vi "Setting2.vi"() -> ()   [LabVIEW 2015]
uses:
  0.Control/Setting_Control_Main Action.ctl
  0.Control/Setting_Control_Pattern Paremeter.ctl
  <vilib>/vision/Measure.llb/Edge Options.ctl
  <vilib>/vision/Measure.llb/Edge Polarity.ctl
  <vilib>/Utility/miscctls.llb/LVPointTypeDef.ctl
  <vilib>/Utility/miscctls.llb/LVBoundsTypeDef.ctl
  <vilib>/userdefined/High Color/IMAQdx.ctl
  <vilib>/vision/NI_Vision_Development_Module.lvlib
panel:
  out "距離(中心到邊)":dbl
  out "間距":sgl
  out "String":string
  out "彈簧距離":sgl
  out "彈簧角度":sgl
  out "塑膠蓋角度":sgl
  out "Pattern":T1(plugin-control)
  in  "相機、光源":T2 {"光源亮度" step=1 scale=0.0..255.0; "相機選擇" items=["相機 1", "相機 2"]; "光源選擇" items=["光源 1", "光源 2"]}
  out "Image":T1(plugin-control)
  in  "Tab Control":enum32{"設定", "Match參數", "找邊參數", "間距參數"}(tab)
  in  "單步測試":bool
  in  "連續測試":bool
  in  "檢測項目塑膠蓋":enum16{"Pattern", "Match", "找邊", "間距"}(ring)
  in  "取像":bool
  in  "連續取像":bool
  in  "離開":bool
  in  "匯入圖片":bool
  in  "確認檢測項目":bool
  in  "樣本比對參數L":T3={"方法"=1, "分數"=800.0, "起始角度"=-5.0, "結束角度"=5.0} {"結束角度" min=-180 max=180 step=5; "方法" items=["快速比對"=1, "精準比對"=2]; "起始角度" min=-180 max=180 step=5}
  in  "pattern_Angle Range":cluster{"Start Angle":sgl, "End Angle":sgl}={"Start Angle"=180.0, "End Angle"=-180.0}
  in  "Scan Direction":u16(ring) items=["Left To Right", "Right To Left", "Top To Bottom", "Bottom To Top"]
  in  "Edge Options":T4={"Edge Polarity"=0, "Kernel Size"=3, "Width"=3, "Minimum Edge Strength"=10.0, "Interpolation Type"=enum."Bilinear Fixed", "Data Processing Method"=enum."Average"} {"Edge Polarity" items=["All Edges", "Rising Edges", "Falling Edges"]; "Minimum Edge Strength" format="%.2f"; "Width" step=2; "Kernel Size" step=2}
  in  "setting":T6={"Contrast"=40, "Filter width"=4, "Steepness"=2, "Subsampling Ratio"=5}
  out "Set action":T7
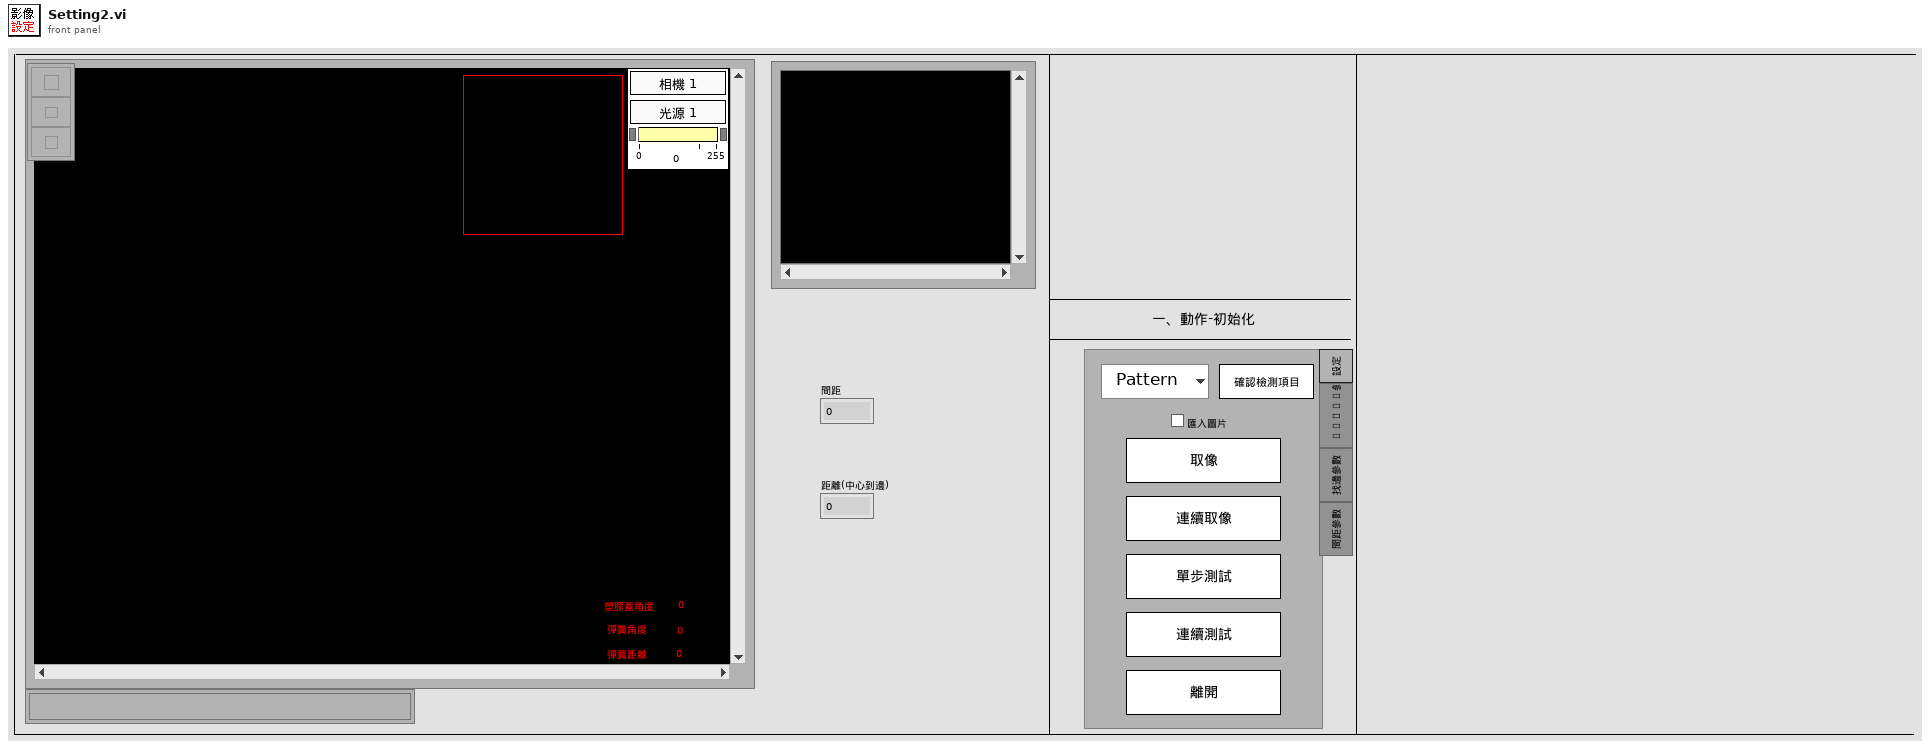
[diagram p1: front panel]
types:
  T1 = typedef "IMAQ Image.ctl" = refnum<image>
  T2 = typedef "Control_Camera&Light.ctl" = cluster{"相機選擇":u8, "光源選擇":u16, "光源亮度":u8}
  T3 = typedef "Setting_Control_Pattern Paremeter.ctl" = cluster{"方法":u16, "分數":sgl, "起始角度":sgl, "結束角度":sgl}
  T4 = typedef "Edge Options.ctl" = cluster{"Edge Polarity":T5, "Kernel Size":u32, "Width":u32, "Minimum Edge Strength":sgl, "Interpolation Type":enum32{"Zero Order", "Bilinear", "Quadratic", "Cubic", "Bilinear Fixed"}, "Data Processing Method":enum32{"Average", "Median"}}
  T5 = typedef "Edge Polarity.ctl" = u32
  T6 = cluster{"Contrast":i32, "Filter width":i32, "Steepness":i32, "Subsampling Ratio":u32}
  T7 = typedef "Setting_Control_Main Action.ctl" = enum16{"一、動作-初始化", "二、動作-單次取像", "三、動作-連續取像", "四、動作-單步測試", "五、動作-連續測試", "六、動作-離開", "1.0 功能-IO控制", "       1.1 IO-初始化", "       1.2 Set Point(EOT On)", "       1.3Set Point(EOT Off)", "       1.4Get Point(SOT)", "2.0功能-相機控制", "       2.1相機-初始化", "       2.2相機-取像", "       2.3相機-關閉", "3.0功能-影像控制", "       3.1影像-初始化", "       3.2影像-更新影像", "       3.3影像-儲存影像", "4.0功能-檢測", "       4.1檢測-初始化", "      4.2浪代-浪代", "             4.2.1浪代-Pattern", "             4.2.2浪代-Match", "             4.2.3檢測-找邊", "             4.2.4檢測-間距", "5.0功能-檔案", "       5.1檔案-初始化", "       5.2檔案-儲存檔案", "       5.3檔案-開啟檔案", "       5.4檔案-匯入檔案", "6.0 錯誤", "7.0等待", "       7.1等待(計算時間)", "8.0離開", "9.0功能-機台驗證", "      9.1機台驗證-初始化", "      9.2機台驗證-檢測", "10.0對話視窗", "11.光源控制", "       11.1光源控制-初始化", "       11.2光源控制-光源開啟", "       11.3光源控制-光源關閉", "       11.4光源控制-通訊關閉"}
  T8 = typedef "LVPointTypeDef.ctl" = cluster{"Horizontal":i16, "Vertical":i16}
  T9 = typedef "IMAQdx.ctl" = refnum<k21>
  T10 = typedef "action_camera.ctl" = enum16{"初始化", "取像", "匯入影像", "結束"}
  T11 = typedef "Control_Indicator Action(FGV).ctl" = enum16{"Set Data", "Get Data", "Idle"}
  T12 = typedef "Image action.ctl" = enum16{"初始化", "創造記憶體", "寫入圖片", "讀取圖片", "刪除圖片", "等待"}
  T13 = typedef "LVBoundsTypeDef.ctl" = cluster{"Width":u32, "Height":u32}
  T14 = typedef "IMAQ Coordinate System" = cluster{"Reference System":cluster{"Origin":cluster{"X":sgl, "Y":sgl}, "Angle (deg)":sgl, "Axis Reference":u32}, "Measurement System":cluster{"Origin":cluster{"X":sgl, "Y":sgl}, "Angle (deg)":sgl, "Axis Reference":u32}}
  T15 = cluster{"樣本比對參數L":T3, "ROI":cluster{"Global Rectangle":i32[], "Contours":cluster{"Contour Type":u32, "ROI Type":u32, "Points":i32[]}[]}, "Coordinate System Out":T14}
  T16 = typedef "Action_Data.ctl" = enum16{"Initialize", "Get Data", "Set Data", "Delete Data", "Idle"}
  T17 = cluster{"setting":cluster{"Contrast":i32, "Filter width":i32, "Steepness":i32, "Subsampling Ratio":u32}, "ROI":cluster{"Global Rectangle":i32[], "Contours":cluster{"Contour Type":u32, "ROI Type":u32, "Points":i32[]}[]}}
  T18 = cluster{"Scan Direction":u16, "ROI":cluster{"Global Rectangle":i32[], "Contours":cluster{"Contour Type":u32, "ROI Type":u32, "Points":i32[]}[]}, "Edge Options":T4}
  T19 = typedef "Control_Indicator(FGV) #.ctl" = cluster{"相機、光源":cluster{"相機選擇":u8, "光源選擇":u16, "光源亮度":u8}, "Session Out":T9, "Cam#Light#Strength":string}
  T20 = typedef "光源通訊_action_control.ctl" = enum16{"initial", "開啟光源", "關閉光源", "close"}
  T21 = typedef "Image Type" = u32
  T22 = cluster{"Global Rectangle":i32[], "Contours":cluster{"Contour Type":u32, "ROI Type":u32, "Points":i32[]}[]}
  T23 = cluster{"Position":cluster{"x":sgl, "y":sgl}, "Angle":sgl, "Scale":sgl, "Score":sgl, "Bounding Box":cluster{"x":sgl, "y":sgl}[]}[]
  T24 = cluster{"Position":cluster{"x":sgl, "y":sgl}, "Angle":sgl, "Scale":sgl, "Score":sgl, "Bounding Box":cluster{"x":sgl, "y":sgl}[]}
  T25 = cluster{"Center (Pixels)":cluster{"X":sgl, "Y":sgl}, "Radius (Pixels)":dbl, "Center (Real-World)":cluster{"X":sgl, "Y":sgl}, "Radius (Real-World)":dbl, "Roundness (Real-World)":dbl, "Average Strength":dbl, "Average SNR (dB)":dbl}
  T26 = cluster{"Search  Direction":u32, "Edge Options":T4, "Show Search Area":bool, "Show Search Lines":bool, "Show Edges Found":bool, "Show Result":bool, "Search Area Color":u32, "Search Lines Color":u32, "Edge Locations Color":u32, "Result Color":u32, "Overlay Group Name":string}
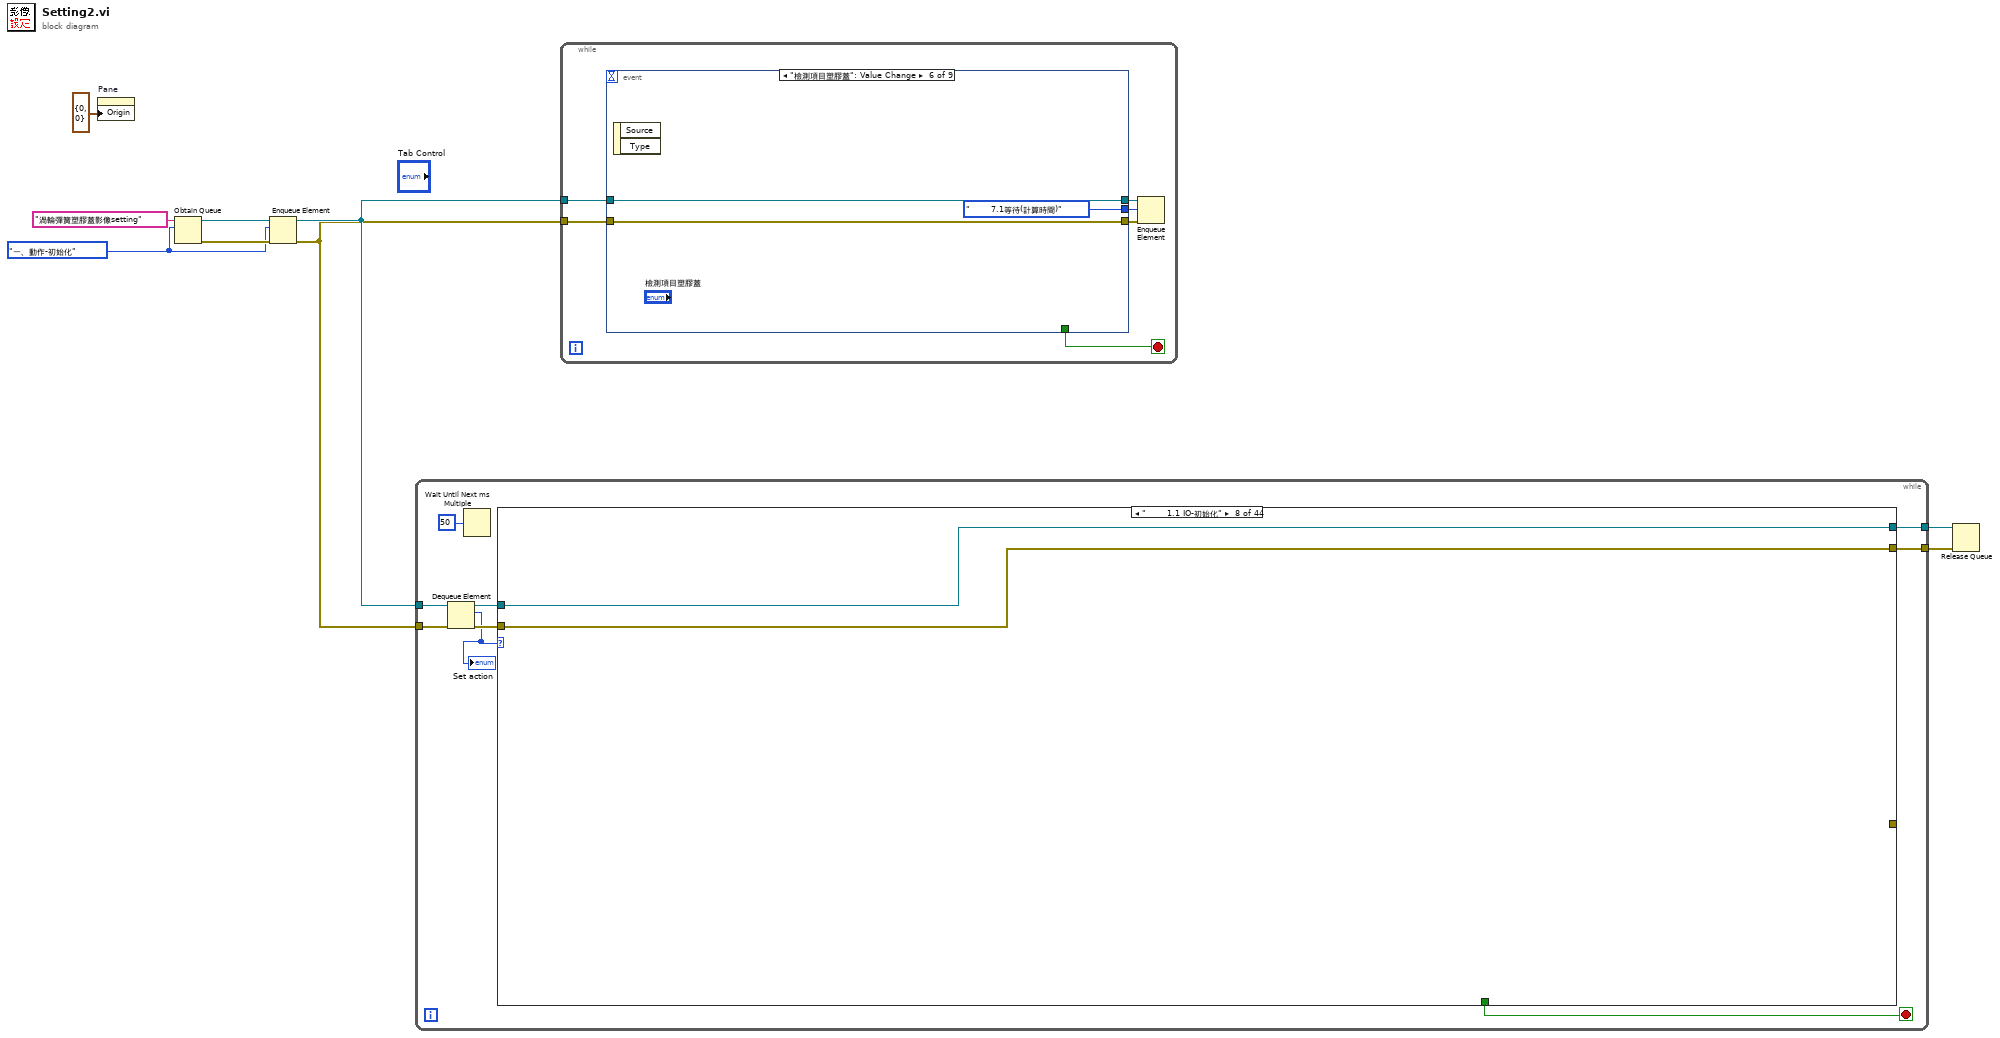
[diagram p0: block diagram]
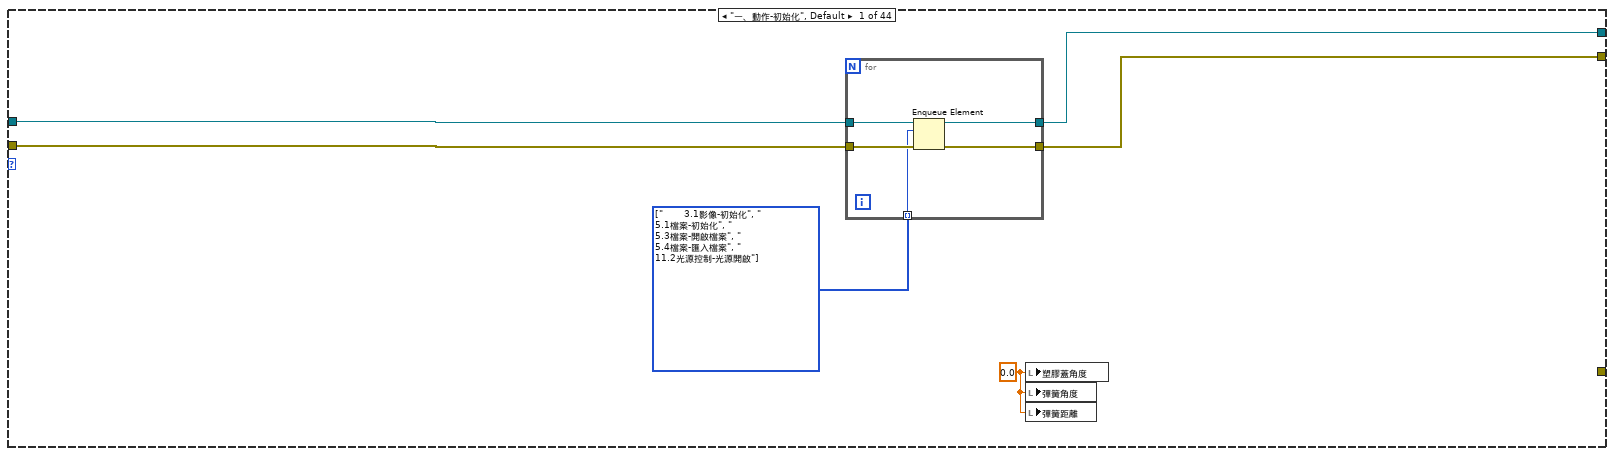
[diagram p2: hidden frame]
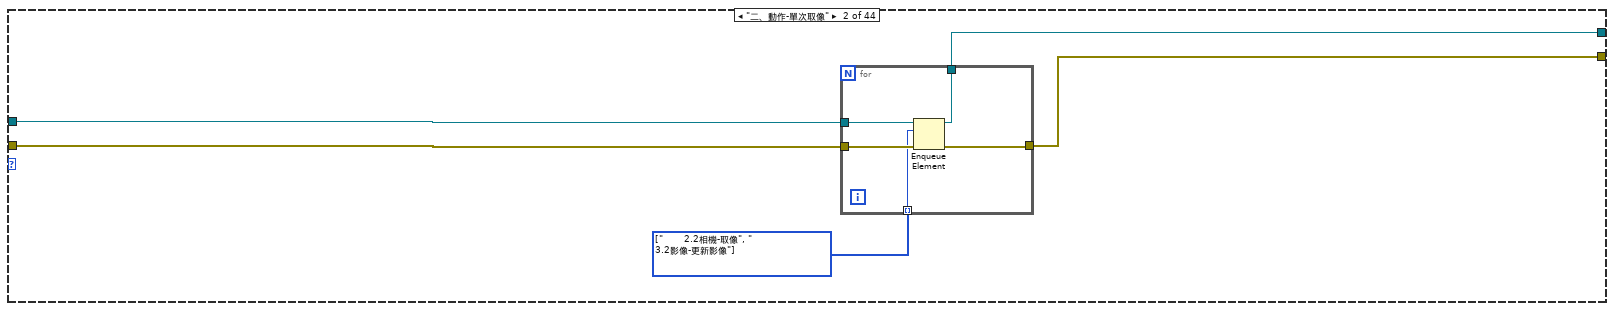
[diagram p3: hidden frame]
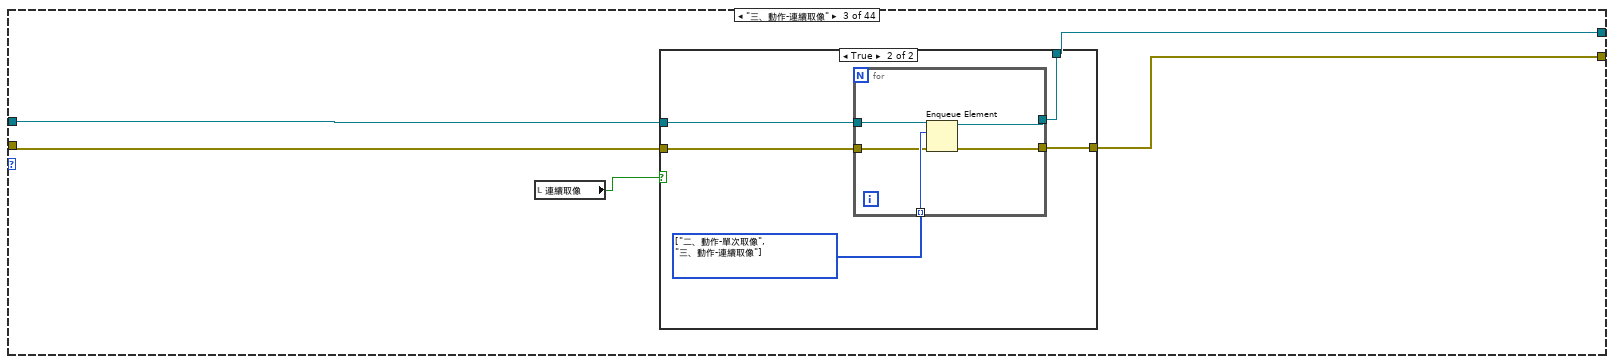
[diagram p4: hidden frame]
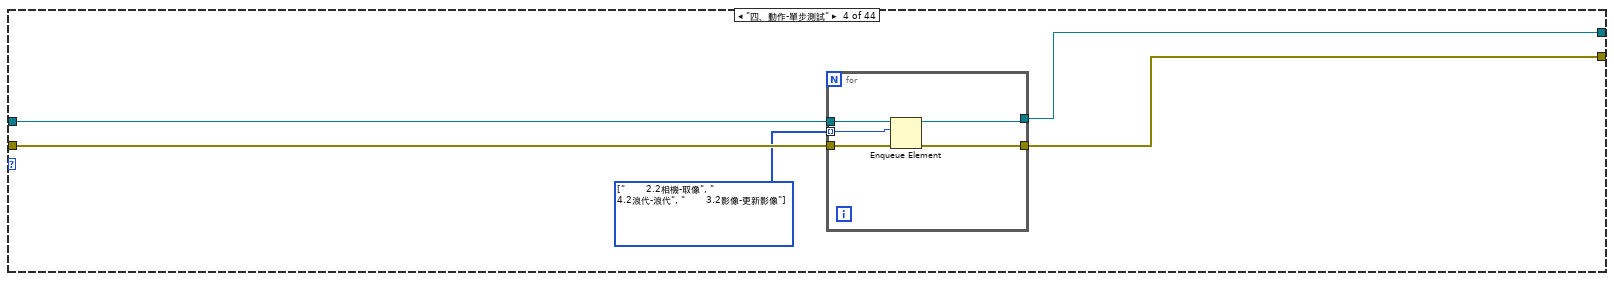
[diagram p6: hidden frame]
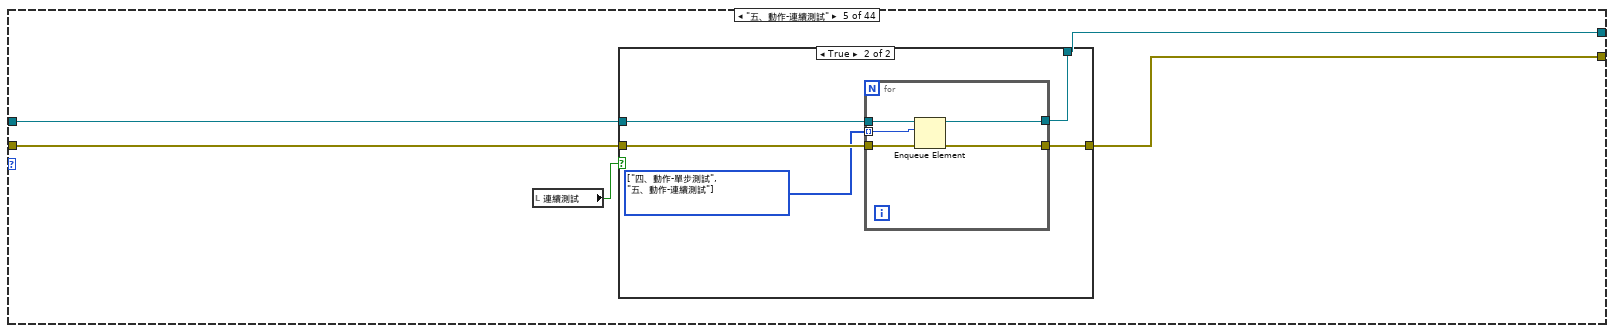
[diagram p7: hidden frame]
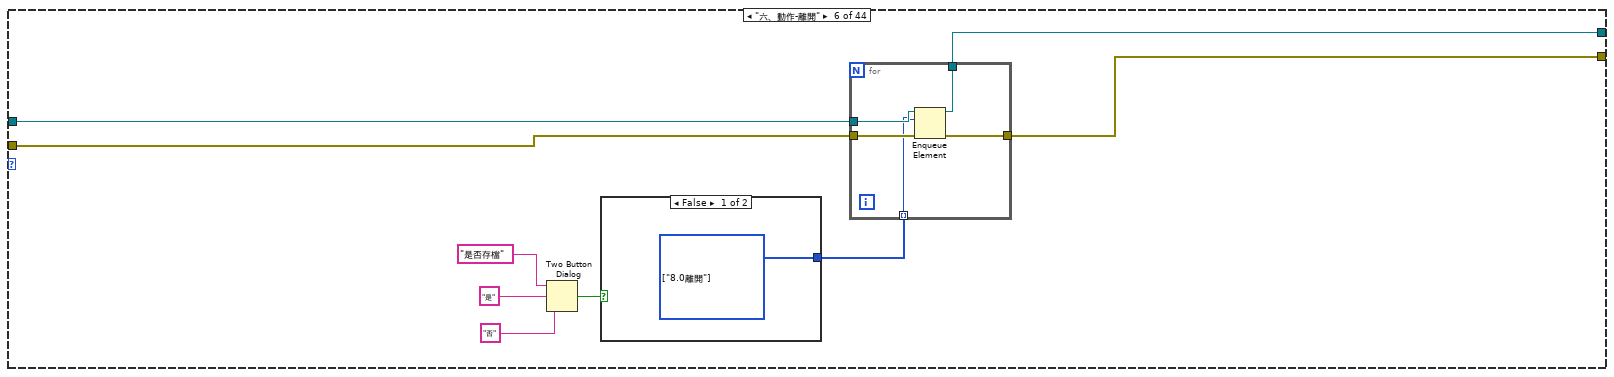
[diagram p9: hidden frame]
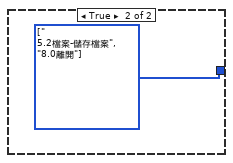
[diagram p10: hidden frame]
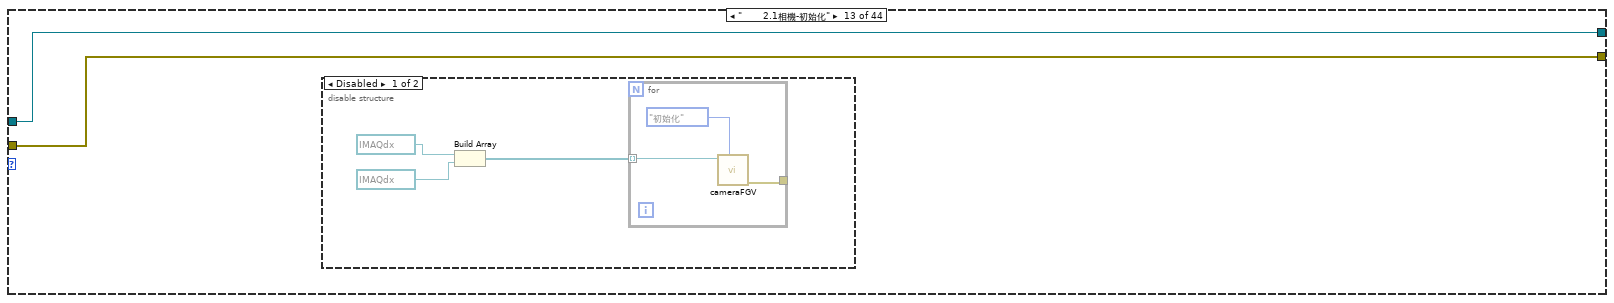
[diagram p16: hidden frame]
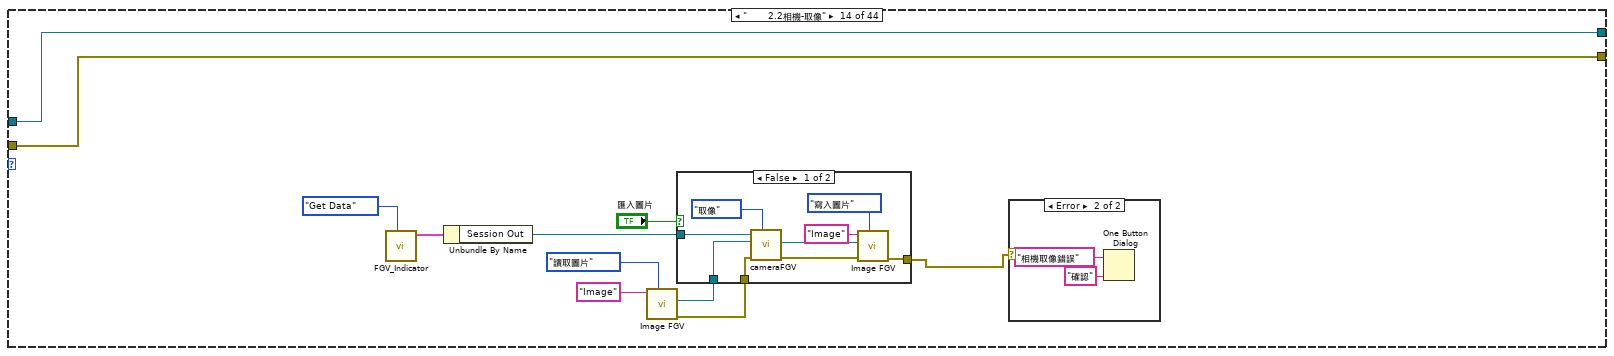
[diagram p18: hidden frame]
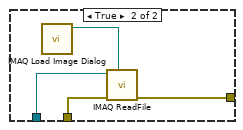
[diagram p20: hidden frame]
diagram:
  w3 = Setting_Control_Main_Action."一、動作-初始化" ("Set action")
  n1 = property on="Pane" class="Pane"("Origin"=T8 {"Horizontal"=0, "Vertical"=0}) -> ()  [unwired: 2 in, 2 out]
  n2 = Obtain Queue(name (unnamed)="渦輪彈簧塑膠蓋影像setting", element data type=w3) -> (queue out=w8:refnum<queue>, error out=w7:errorcluster)  [unwired: 3 in, 1 out]
  n3 = Enqueue Element(queue=w8, element=w3, error in (no error)=w7) -> (queue out=w6:refnum<queue>, error out=w5:errorcluster)  [unwired: 1 in, 1 out]
  n4 = while {
    tunnel: w6 -> [w18]
    tunnel: w5 -> [w17]
    tunnel: [w11] -> w2
    tunnel: [w10] -> w1
    stop <- w16 stop-if-true
    n5 = Dequeue Element(queue=w18, error in (no error)=w17) -> (queue out=w15:refnum<queue>, element=w12:T7, error out=w14:errorcluster)  [unwired: 1 in, 1 out]
    "Set action" <- w12
    n6 = Wait Until Next ms Multiple(millisecond multiple=u32 50) -> ()  [unwired: 1 out]
    n7 = case shown="\"       1.1 IO-初始化\"" w12 {
      tunnel: [_ _ _ _ _ _ _ _ _ _ _ _ _ _ _ _ _ _ _ _ _ _ _ _ _ _ _ _ _ _ _ _ _ _ TRUE _ _ _ _ _ _ _ _ _] -> w16
      tunnel: w15 -> [w21 w34 w44 w61 w71 w92 w101 w103 w105 w107 w109 w111 w113 w126 w147 w155 w160 w183 w188 w190 w192 w195 w357 w381 w409 w435 w448 w451 w474 w493 w564 w579 w581 w583 w586 w588 w590 w592 w594 w596 w598 w612 w624 w628]
      tunnel: w14 -> [w24 w33 w43 w60 w70 w91 w100 w102 w104 w106 w108 w110 w112 w121 w146 w154 w158 w177 w187 w189 w191 w194 w355 w379 w408 w434 w447 w449 w473 w492 w563 w578 w580 w582 w585 w587 w589 w591 w593 w595 w597 w611 w623 w627]
      tunnel: [w22 w31 w42 w59 w69 w90 w101 w103 w105 w107 w109 w111 w113 w126 w147 w155 w160 w183 w188 w190 w192 w195 w356 w380 w407 w433 w448 w451 w474 w494 w564 w579 w581 w583 w586 w588 w590 w592 w594 w596 w598 w612 w624 w628] -> w11
      tunnel: [w23 w32 w41 w58 w68 w89 w100 w102 w104 w106 w108 w110 w112 w121 w146 w154 w157 w175 w187 w189 w191 w194 w354 w378 w406 w432 w447 w449 w473 w491 w563 w578 w580 w582 w585 w587 w589 w591 w593 w595 w597 w611 w623 w627] -> w10
      tunnel: [_ _ _ _ _ _ _ _ _ _ _ _ _ _ _ _ _ _ _ _ _ w193 _ _ _ _ _ _ _ w489 _ _ _ _ _ _ _ _ _ _ _ _ _ _] -> _
      frame "一、動作-初始化", Default {
        w19 = sgl 0.0 ("塑膠蓋角度")
        w20 = T7[] [enum."       3.1影像-初始化", enum."       5.1檔案-初始化", enum."       5.3檔案-開啟檔案", enum."       5.4檔案-匯入檔案", enum."       11.2光源控制-光源開啟"] items=["一、動作-初始化", "二、動作-單次取像", "三、動作-連續取像", "四、動作-單步測試", "五、動作-連續測試", "六、動作-離開", "1.0 功能-IO控制", "       1.1 IO-初始化", "       1.2 Set Point(EOT On)", "       1.3Set Point(EOT Off)", "       1.4Get Point(SOT)", "2.0功能-相機控制", "       2.1相機-初始化", "       2.2相機-取像", "       2.3相機-關閉", "3.0功能-影像控制", "       3.1影像-初始化", "       3.2影像-更新影像", "       3.3影像-儲存影像", "4.0功能-檢測", "       4.1檢測-初始化", "      4.2浪代-浪代", "             4.2.1浪代-Pattern", "             4.2.2浪代-Match", "             4.2.3檢測-找邊", "             4.2.4檢測-間距", "5.0功能-檔案", "       5.1檔案-初始化", "       5.2檔案-儲存檔案", "       5.3檔案-開啟檔案", "       5.4檔案-匯入檔案", "6.0 錯誤", "7.0等待", "       7.1等待(計算時間)", "8.0離開", "9.0功能-機台驗證", "      9.1機台驗證-初始化", "      9.2機台驗證-檢測", "10.0對話視窗", "11.光源控制", "       11.1光源控制-初始化", "       11.2光源控制-光源開啟", "       11.3光源控制-光源關閉", "       11.4光源控制-通訊關閉"]
        n8 = for {
          tunnel: w21 -> [w29]
          tunnel: w24 -> [w28]
          tunnel: [w27] -> w23
          tunnel: [w26] -> w22
          tunnel: w20 -> [w25] mode=indexing
          n9 = Enqueue Element(queue=w29, element=w25, error in (no error)=w28) -> (queue out=w26:refnum<queue>, error out=w27:errorcluster)  [unwired: 1 in, 1 out]
        }
        n10 = local write "塑膠蓋角度"(w19) -> ()
        n11 = local write "彈簧角度"(w19) -> ()
        n12 = local write "彈簧距離"(w19) -> ()
      }
      frame "二、動作-單次取像" {
        w30 = T7[] [enum."       2.2相機-取像", enum."       3.2影像-更新影像"] items=["一、動作-初始化", "二、動作-單次取像", "三、動作-連續取像", "四、動作-單步測試", "五、動作-連續測試", "六、動作-離開", "1.0 功能-IO控制", "       1.1 IO-初始化", "       1.2 Set Point(EOT On)", "       1.3Set Point(EOT Off)", "       1.4Get Point(SOT)", "2.0功能-相機控制", "       2.1相機-初始化", "       2.2相機-取像", "       2.3相機-關閉", "3.0功能-影像控制", "       3.1影像-初始化", "       3.2影像-更新影像", "       3.3影像-儲存影像", "4.0功能-檢測", "       4.1檢測-初始化", "      4.2浪代-浪代", "             4.2.1浪代-Pattern", "             4.2.2浪代-Match", "             4.2.3檢測-找邊", "             4.2.4檢測-間距", "5.0功能-檔案", "       5.1檔案-初始化", "       5.2檔案-儲存檔案", "       5.3檔案-開啟檔案", "       5.4檔案-匯入檔案", "6.0 錯誤", "7.0等待", "       7.1等待(計算時間)", "8.0離開", "9.0功能-機台驗證", "      9.1機台驗證-初始化", "      9.2機台驗證-檢測", "10.0對話視窗", "11.光源控制", "       11.1光源控制-初始化", "       11.2光源控制-光源開啟", "       11.3光源控制-光源關閉", "       11.4光源控制-通訊關閉"]
        n13 = for {
          tunnel: w34 -> [w39]
          tunnel: w33 -> [w38]
          tunnel: [w37] -> w32
          tunnel: [w36] -> w31
          tunnel: w30 -> [w35] mode=indexing
          n14 = Enqueue Element(queue=w39, element=w35, error in (no error)=w38) -> (queue out=w36:refnum<queue>, error out=w37:errorcluster)  [unwired: 1 in, 1 out]
        }
      }
      frame "三、動作-連續取像" {
        n15 = local read "連續取像"() -> (w40:bool)
        n16 = case shown="True" w40 {
          tunnel: w44 -> [w46 w50]
          tunnel: w43 -> [w45 w49]
          tunnel: [w46 w48] -> w42
          tunnel: [w45 w47] -> w41
          frame False {
          }
          frame True {
            w51 = T7[] [enum."二、動作-單次取像", enum."三、動作-連續取像"] items=["一、動作-初始化", "二、動作-單次取像", "三、動作-連續取像", "四、動作-單步測試", "五、動作-連續測試", "六、動作-離開", "1.0 功能-IO控制", "       1.1 IO-初始化", "       1.2 Set Point(EOT On)", "       1.3Set Point(EOT Off)", "       1.4Get Point(SOT)", "2.0功能-相機控制", "       2.1相機-初始化", "       2.2相機-取像", "       2.3相機-關閉", "3.0功能-影像控制", "       3.1影像-初始化", "       3.2影像-更新影像", "       3.3影像-儲存影像", "4.0功能-檢測", "       4.1檢測-初始化", "      4.2浪代-浪代", "             4.2.1浪代-Pattern", "             4.2.2浪代-Match", "             4.2.3檢測-找邊", "             4.2.4檢測-間距", "5.0功能-檔案", "       5.1檔案-初始化", "       5.2檔案-儲存檔案", "       5.3檔案-開啟檔案", "       5.4檔案-匯入檔案", "6.0 錯誤", "7.0等待", "       7.1等待(計算時間)", "8.0離開", "9.0功能-機台驗證", "      9.1機台驗證-初始化", "      9.2機台驗證-檢測", "10.0對話視窗", "11.光源控制", "       11.1光源控制-初始化", "       11.2光源控制-光源開啟", "       11.3光源控制-光源關閉", "       11.4光源控制-通訊關閉"]
            n17 = for {
              tunnel: [w56] -> w47
              tunnel: [w55] -> w48
              tunnel: w51 -> [w54] mode=indexing
              tunnel: w50 -> [w53]
              tunnel: w49 -> [w52]
              n18 = Enqueue Element(queue=w53, element=w54, error in (no error)=w52) -> (queue out=w55:refnum<queue>, error out=w56:errorcluster)  [unwired: 1 in, 1 out]
            }
          }
        }
      }
      frame "四、動作-單步測試" {
        w57 = T7[] [enum."       2.2相機-取像", enum."      4.2浪代-浪代", enum."       3.2影像-更新影像"] items=["一、動作-初始化", "二、動作-單次取像", "三、動作-連續取像", "四、動作-單步測試", "五、動作-連續測試", "六、動作-離開", "1.0 功能-IO控制", "       1.1 IO-初始化", "       1.2 Set Point(EOT On)", "       1.3Set Point(EOT Off)", "       1.4Get Point(SOT)", "2.0功能-相機控制", "       2.1相機-初始化", "       2.2相機-取像", "       2.3相機-關閉", "3.0功能-影像控制", "       3.1影像-初始化", "       3.2影像-更新影像", "       3.3影像-儲存影像", "4.0功能-檢測", "       4.1檢測-初始化", "      4.2浪代-浪代", "             4.2.1浪代-Pattern", "             4.2.2浪代-Match", "             4.2.3檢測-找邊", "             4.2.4檢測-間距", "5.0功能-檔案", "       5.1檔案-初始化", "       5.2檔案-儲存檔案", "       5.3檔案-開啟檔案", "       5.4檔案-匯入檔案", "6.0 錯誤", "7.0等待", "       7.1等待(計算時間)", "8.0離開", "9.0功能-機台驗證", "      9.1機台驗證-初始化", "      9.2機台驗證-檢測", "10.0對話視窗", "11.光源控制", "       11.1光源控制-初始化", "       11.2光源控制-光源開啟", "       11.3光源控制-光源關閉", "       11.4光源控制-通訊關閉"]
        n19 = for {
          tunnel: w61 -> [w66]
          tunnel: w60 -> [w65]
          tunnel: [w64] -> w59
          tunnel: [w63] -> w58
          tunnel: w57 -> [w62] mode=indexing
          n20 = Enqueue Element(queue=w66, element=w62, error in (no error)=w65) -> (queue out=w64:refnum<queue>, error out=w63:errorcluster)  [unwired: 1 in, 1 out]
        }
      }
      frame "五、動作-連續測試" {
        n21 = local read "連續測試"() -> (w67:bool)
        n22 = case shown="True" w67 {
          tunnel: w71 -> [w73 w78]
          tunnel: w70 -> [w72 w77]
          tunnel: [w73 w76] -> w69
          tunnel: [w72 w75] -> w68
          frame False {
          }
          frame True {
            w74 = T7[] [enum."四、動作-單步測試", enum."五、動作-連續測試"] items=["一、動作-初始化", "二、動作-單次取像", "三、動作-連續取像", "四、動作-單步測試", "五、動作-連續測試", "六、動作-離開", "1.0 功能-IO控制", "       1.1 IO-初始化", "       1.2 Set Point(EOT On)", "       1.3Set Point(EOT Off)", "       1.4Get Point(SOT)", "2.0功能-相機控制", "       2.1相機-初始化", "       2.2相機-取像", "       2.3相機-關閉", "3.0功能-影像控制", "       3.1影像-初始化", "       3.2影像-更新影像", "       3.3影像-儲存影像", "4.0功能-檢測", "       4.1檢測-初始化", "      4.2浪代-浪代", "             4.2.1浪代-Pattern", "             4.2.2浪代-Match", "             4.2.3檢測-找邊", "             4.2.4檢測-間距", "5.0功能-檔案", "       5.1檔案-初始化", "       5.2檔案-儲存檔案", "       5.3檔案-開啟檔案", "       5.4檔案-匯入檔案", "6.0 錯誤", "7.0等待", "       7.1等待(計算時間)", "8.0離開", "9.0功能-機台驗證", "      9.1機台驗證-初始化", "      9.2機台驗證-檢測", "10.0對話視窗", "11.光源控制", "       11.1光源控制-初始化", "       11.2光源控制-光源開啟", "       11.3光源控制-光源關閉", "       11.4光源控制-通訊關閉"]
            n23 = for {
              tunnel: w78 -> [w83]
              tunnel: w77 -> [w82]
              tunnel: [w81] -> w76
              tunnel: [w80] -> w75
              tunnel: w74 -> [w79] mode=indexing
              n24 = Enqueue Element(queue=w83, element=w79, error in (no error)=w82) -> (queue out=w81:refnum<queue>, error out=w80:errorcluster)  [unwired: 1 in, 1 out]
            }
          }
        }
      }
      frame "六、動作-離開" {
        n25 = Two Button Dialog(message="是否存檔", 1:"否" ("F button name (\"Cancel\")"), 2:"是" ("T button name (\"OK\")")) -> (T button?=w88:bool)
        n26 = case shown="False" w88 {
          tunnel: [w93 w94] -> w84
          frame False {
            w93 = T7[] [enum."8.0離開"] items=["一、動作-初始化", "二、動作-單次取像", "三、動作-連續取像", "四、動作-單步測試", "五、動作-連續測試", "六、動作-離開", "1.0 功能-IO控制", "       1.1 IO-初始化", "       1.2 Set Point(EOT On)", "       1.3Set Point(EOT Off)", "       1.4Get Point(SOT)", "2.0功能-相機控制", "       2.1相機-初始化", "       2.2相機-取像", "       2.3相機-關閉", "3.0功能-影像控制", "       3.1影像-初始化", "       3.2影像-更新影像", "       3.3影像-儲存影像", "4.0功能-檢測", "       4.1檢測-初始化", "      4.2浪代-浪代", "             4.2.1浪代-Pattern", "             4.2.2浪代-Match", "             4.2.3檢測-找邊", "             4.2.4檢測-間距", "5.0功能-檔案", "       5.1檔案-初始化", "       5.2檔案-儲存檔案", "       5.3檔案-開啟檔案", "       5.4檔案-匯入檔案", "6.0 錯誤", "7.0等待", "       7.1等待(計算時間)", "8.0離開", "9.0功能-機台驗證", "      9.1機台驗證-初始化", "      9.2機台驗證-檢測", "10.0對話視窗", "11.光源控制", "       11.1光源控制-初始化", "       11.2光源控制-光源開啟", "       11.3光源控制-光源關閉", "       11.4光源控制-通訊關閉"]
          }
          frame True {
            w94 = T7[] [enum."       5.2檔案-儲存檔案", enum."8.0離開"] items=["一、動作-初始化", "二、動作-單次取像", "三、動作-連續取像", "四、動作-單步測試", "五、動作-連續測試", "六、動作-離開", "1.0 功能-IO控制", "       1.1 IO-初始化", "       1.2 Set Point(EOT On)", "       1.3Set Point(EOT Off)", "       1.4Get Point(SOT)", "2.0功能-相機控制", "       2.1相機-初始化", "       2.2相機-取像", "       2.3相機-關閉", "3.0功能-影像控制", "       3.1影像-初始化", "       3.2影像-更新影像", "       3.3影像-儲存影像", "4.0功能-檢測", "       4.1檢測-初始化", "      4.2浪代-浪代", "             4.2.1浪代-Pattern", "             4.2.2浪代-Match", "             4.2.3檢測-找邊", "             4.2.4檢測-間距", "5.0功能-檔案", "       5.1檔案-初始化", "       5.2檔案-儲存檔案", "       5.3檔案-開啟檔案", "       5.4檔案-匯入檔案", "6.0 錯誤", "7.0等待", "       7.1等待(計算時間)", "8.0離開", "9.0功能-機台驗證", "      9.1機台驗證-初始化", "      9.2機台驗證-檢測", "10.0對話視窗", "11.光源控制", "       11.1光源控制-初始化", "       11.2光源控制-光源開啟", "       11.3光源控制-光源關閉", "       11.4光源控制-通訊關閉"]
          }
        }
        n27 = for {
          tunnel: w92 -> [w99]
          tunnel: w91 -> [w98]
          tunnel: [w97] -> w90
          tunnel: [w96] -> w89
          tunnel: w84 -> [w95] mode=indexing
          n28 = Enqueue Element(queue=w99, element=w95, error in (no error)=w98) -> (queue out=w97:refnum<queue>, error out=w96:errorcluster)  [unwired: 1 in, 1 out]
        }
      }
      frame "1.0 功能-IO控制" {
      }
      frame "       1.1 IO-初始化" {
      }
      frame "       1.2 Set Point(EOT On)" {
      }
      frame "       1.3Set Point(EOT Off)" {
      }
      frame "       1.4Get Point(SOT)" {
      }
      frame "2.0功能-相機控制" {
      }
      frame "       2.1相機-初始化" {
        n29 = disable-structure shown="Disabled" {
          frame Disabled {
            n30 = Build Array(T9 "cam0" ("Session In"), T9 "cam1" ("Session In")) -> (w114:T9[])
            n31 = for {
              tunnel: w114 -> [w118] mode=indexing
              tunnel: [w117] -> _
              n32 = call "cameraFGV.vi"("action_camera"=action_camera."初始化", "Session In"=w118) -> ("error constant 2"=w117:errorcluster)  [unwired: 7 in, 2 out]
            }
          }
          frame Enabled {
          }
        }
      }
      frame "       2.2相機-取像" {
        n33 = call "FGV_Indicator.vi"("Action"=Control_Indicator_Action(FGV)."Get Data") -> ("Indicator Data Out"=w122:T19)  [unwired: 10 in]
        n34 = Unbundle By Name(w122) -> ("Session Out"=w124:T9)
        n35 = call "Image FGV.vi"("Image action"=Image_action."讀取圖片", "圖片名稱"="Image") -> ("error out"=w127:errorcluster, "Image Out"=w128:T1)  [unwired: 8 in]
        n36 = case shown="False" "匯入圖片" {
          tunnel: w128 -> [w141 w145]
          tunnel: w127 -> [w140 w144]
          tunnel: w124 -> [w136 _]
          tunnel: [w135 w142] -> w120
          frame False {
            n37 = call "cameraFGV.vi"("action_camera"=action_camera."取像", "error constant"=w140, "Image In"=w141, "Session In"=w136) -> ("error constant 2"=w139:errorcluster, "Image Out"=w138:T1)  [unwired: 5 in, 1 out]
            n38 = call "Image FGV.vi"("Image action"=Image_action."寫入圖片", "error in (no error)"=w139, "Image In"=w138, "圖片名稱"="Image") -> ("error out"=w135:errorcluster)  [unwired: 6 in, 1 out]
          }
          frame True {
            n39 = call "IMAQ Load Image Dialog"() -> ("Path"=w143:path)  [unwired: 9 in, 2 out]
            n40 = call "IMAQ ReadFile"("File Path"=w143, "error in (no error)"=w144, "Image"=w145) -> ("error out"=w142:errorcluster)  [unwired: 4 in, 4 out]
          }
        }
        n41 = case shown="Error" w120 {
          frame No Error {
          }
          frame Error {
            n42 = One Button Dialog(message="相機取像錯誤", button name ("OK")="確認") -> ()  [unwired: 1 out]
          }
        }
      }
      frame "       2.3相機-關閉" {
        n43 = disable-structure shown="Disabled" {
          frame Disabled {
            n44 = Build Array(T9 "cam0" ("Session In"), T9 "cam1" ("Session In")) -> (w148:T9[])
            n45 = for {
              tunnel: w148 -> [w152] mode=indexing
              tunnel: [w151] -> _
              n46 = call "cameraFGV.vi"("action_camera"=action_camera."結束", "Session In"=w152) -> ("error constant 2"=w151:errorcluster)  [unwired: 7 in, 2 out]
            }
          }
          frame Enabled {
          }
        }
      }
      frame "3.0功能-影像控制" {
      }
      frame "       3.1影像-初始化" {
        n47 = disable-structure shown="Enabled" {
          disable-tunnel: w158 -> [w162 w172]
          disable-tunnel: [w161 w172] -> w157
          frame Enabled {
            w163 = T21[] [0, 0] items=["Grayscale (U8)", "Grayscale (I16)", "Grayscale (SGL)", "Complex (CSG)", "RGB (U32)", "HSL (U32)", "RGB (U64)", "Grayscale (U16)"]
            n48 = call "Image FGV.vi"("Image action"=Image_action."初始化", "error in (no error)"=w162) -> ("error out"=w165:errorcluster)  [unwired: 8 in, 1 out]
            n49 = for {
              tunnel: w165 -> [w171]
              tunnel: string[] ["Image", "Pattern"] -> [w169] mode=indexing
              tunnel: w163 -> [w168] mode=indexing
              tunnel: [w167] -> w161
              n50 = call "Image FGV.vi"("Image action"=Image_action."創造記憶體", "error in (no error)"=w171, "Image Type"=w168, "圖片名稱"=w169) -> ("error out"=w167:errorcluster)  [unwired: 6 in, 1 out]
            }
          }
          frame Disabled {
          }
        }
        n51 = property on="Image" class="ImageControl"("Zoom to Fit Mode"=TRUE) -> ()  [unwired: 2 in, 2 out]
        n52 = property on="Pattern" class="ImageControl"("Zoom to Fit Mode"=TRUE) -> ()  [unwired: 2 in, 2 out]
      }
      frame "       3.2影像-更新影像" {
        n53 = call "Image FGV.vi"("Image action"=Image_action."讀取圖片", "error in (no error)"=w177, "圖片名稱"="Image") -> ("error out"=w176:errorcluster, "Image Out"=w174:T1)  [unwired: 7 in]
        n54 = disable-structure shown="Enabled" {
          disable-tunnel: w174 -> [w185 w186]
          disable-tunnel: [w184 w186] -> w173
          frame Disabled {
            n55 = call "點檢_VI_畫十字線.vi"("Refnum in"=w185) -> ("Refnum out"=w184:T1)  [unwired: 8 in, 2 out]
          }
          frame Enabled {
          }
        }
        "Image" <- w173
        n56 = call "Image FGV.vi"("Image action"=Image_action."讀取圖片", "error in (no error)"=w176, "圖片名稱"="Pattern") -> ("error out"=w175:errorcluster, "Image Out"=→"Pattern":T1)  [unwired: 7 in]
      }
      frame "       3.3影像-儲存影像" {
      }
      frame "4.0功能-檢測" {
      }
      frame "       4.1檢測-初始化" {
      }
      frame "      4.2浪代-浪代" {
        n57 = disable-structure shown="Enabled" {
          disable-tunnel: [w215 _] -> w193
          frame Enabled {
            n58 = call "FGV_Indicator.vi"("Action"=Control_Indicator_Action(FGV)."Get Data") -> ("Indicator Data Out"=w211:T19)  [unwired: 10 in]
            n59 = Unbundle By Name(w211) -> ("相機、光源"=w210:cluster{"相機選擇":u8, "光源選擇":u16, "光源亮度":u8})
            n60 = property on="檢測項目塑膠蓋" class="Enum (strict)"() -> ("Strings []"=w214:string[])  [unwired: 2 in, 2 out]
            n61 = Unbundle By Name(w210) -> ("相機選擇"=w207:u8)
            n62 = To Long Integer(number=enum16{"Pattern", "Match", "找邊", "找圓"}."Match" ("檢測項目塑膠蓋 2")) -> (32bit integer=w212:i32)
            n63 = Index Array(array=w214, index=w212) -> (element=w208:string)
            n64 = case shown="1" w207 {
              tunnel: w207 -> [w224 w298]
              tunnel: w208 -> [w223 w296]
              tunnel: [_ w252] -> w215
              tunnel: [w217 w249] -> w199
              tunnel: [w216 w247] -> w198
              frame 0, Default {
                w236 = u16 1 items=["Find Reference", "Update CoordSys"] ("Mode")
                n65 = Number To Decimal String(number=w224) -> (decimal integer string=w221:string)  [unwired: 1 in]
                n66 = Concatenate Strings(w223, "-" ("string"), w221) -> (w222:string)
                n67 = call "Main_FGV_Data.vi"("Action_Data"=Action_Data."Get Data", "Data name"=w222) -> ("Data  Out"=w233:cluster{"Data name":string, "Data":variant})  [unwired: 8 in, 1 out]
                n68 = Unbundle By Name(w233) -> ("Data"=w232:variant)
                n69 = Variant To Data(type=T15 {"樣本比對參數L"={"方法"=0, "分數"=0.0, "起始角度"=0.0, "結束角度"=0.0}, "ROI"={"Global Rectangle"=[], "Contours"=[]}, "Coordinate System Out"={"Reference System"={"Origin"={"X"=0.0, "Y"=0.0}, "Angle (deg)"=0.0, "Axis Reference"=0}, "Measurement System"={"Origin"={"X"=0.0, "Y"=0.0}, "Angle (deg)"=0.0, "Axis Reference"=0}}} ("output cluster"), Variant=w232) -> (data=w230:T15, error out=w219:errorcluster)  [unwired: 1 in]
                n70 = call "Image FGV.vi"("Image action"=Image_action."讀取圖片", "圖片名稱"="Pattern") -> ("Image Out"=w235:T1)  [unwired: 8 in, 1 out]
                n71 = call "Image FGV.vi"("Image action"=Image_action."讀取圖片", "圖片名稱"="Image") -> ("Image Out"=w237:T1)  [unwired: 8 in, 1 out]
                n72 = Unbundle(w230) -> ("樣本比對參數L"=w218:T3, "ROI"=w229:T22, "Coordinate System Out"=w228:T14)
                n73 = call "浪代_Match_Sub.vi"("樣本比對參數"=w218, "ROI Descriptor"=w229, "Mode"=w236, "error in (no error)"=w219, "Coordinate System In"=w228, "Template Image"=w235, "Image"=w237) -> ("Matches (real-world)"=w227:T23)  [unwired: 1 in, 3 out]
                n74 = Index Array(array=w227) -> (element=w226:T24)  [unwired: 1 in]
                n75 = Unbundle By Name(w218) -> ("分數"=w216:sgl)
                n76 = Unbundle By Name(w226) -> ("Angle"=→"塑膠蓋角度":sgl, "Score"=w217:sgl)
              }
              frame 1 {
                w273 = u16 1 items=["Find Reference", "Update CoordSys"] ("Mode")
                n77 = Number To Decimal String(number=w298) -> (decimal integer string=w295:string)  [unwired: 1 in]
                n78 = disable-structure shown="Enabled" {
                  disable-tunnel: ["找圓" ("string") "間距" ("element")] -> w292
                  frame Disabled {
                  }
                  frame Enabled {
                  }
                }
                n79 = Concatenate Strings(w296, "-" ("string"), w295) -> (w294:string)
                n80 = Build Array(w294, "找邊" ("string"), w292) -> (w289:string[])
                n81 = for {
                  tunnel: w289 -> [w333] mode=indexing
                  tunnel: [w332] -> w285 mode=indexing
                  n82 = call "Main_FGV_Data.vi"("Action_Data"=Action_Data."Get Data", "Data name"=w333) -> ("Data  Out"=w332:cluster{"Data name":string, "Data":variant})  [unwired: 8 in, 1 out]
                }
                n83 = Index Array(array=w285, index #1=0 ("index"), index #2=1 ("index"), index #3=2 ("index")) -> (element #1=w284:cluster{"Data name":string, "Data":variant}, element #2=w283:cluster{"Data name":string, "Data":variant}, element #3=w282:cluster{"Data name":string, "Data":variant})
                n84 = Unbundle By Name(w284) -> ("Data"=w291:variant)
                n85 = Unbundle By Name(w283) -> ("Data"=w281:variant)
                n86 = Unbundle By Name(w282) -> ("Data"=w280:variant)
                n87 = Variant To Data(type=T15 {"樣本比對參數L"={"方法"=0, "分數"=0.0, "起始角度"=0.0, "結束角度"=0.0}, "ROI"={"Global Rectangle"=[], "Contours"=[]}, "Coordinate System Out"={"Reference System"={"Origin"={"X"=0.0, "Y"=0.0}, "Angle (deg)"=0.0, "Axis Reference"=0}, "Measurement System"={"Origin"={"X"=0.0, "Y"=0.0}, "Angle (deg)"=0.0, "Axis Reference"=0}}} ("output cluster"), Variant=w291) -> (data=w269:T15, error out=w264:errorcluster)  [unwired: 1 in]
                n88 = Variant To Data(type=T17 {"setting"={"Contrast"=0, "Filter width"=0, "Steepness"=0, "Subsampling Ratio"=0}, "ROI"={"Global Rectangle"=[], "Contours"=[]}} ("output cluster"), Variant=w280) -> (data=w259:T17, error out=w262:errorcluster)  [unwired: 1 in]
                n89 = Variant To Data(type=T18 {"Scan Direction"=0, "ROI"={"Global Rectangle"=[], "Contours"=[]}, "Edge Options"={"Edge Polarity"=0, "Kernel Size"=0, "Width"=0, "Minimum Edge Strength"=0.0, "Interpolation Type"=enum."Zero Order", "Data Processing Method"=enum."Average"}} ("output cluster"), Variant=w281) -> (data=w260:T18, error out=w263:errorcluster)  [unwired: 1 in]
                n90 = Merge Errors(w264, w263, w262) -> (w261:errorcluster)
                n91 = Unbundle(w269) -> ("樣本比對參數L"=w248:T3, "ROI"=w268:T22, "Coordinate System Out"=w267:T14)
                n92 = Unbundle(w260) -> ("Scan Direction"=w257:u16, "ROI"=w256:T22, "Edge Options"=w255:T4)
                n93 = call "Image FGV.vi"("Image action"=Image_action."讀取圖片", "圖片名稱"="Pattern") -> ("Image Out"=w278:T1)  [unwired: 8 in, 1 out]
                n94 = call "Image FGV.vi"("Image action"=Image_action."讀取圖片", "圖片名稱"="Image") -> ("Image Out"=w254:T1)  [unwired: 8 in, 1 out]
                n95 = call "浪代_Match_Sub.vi"("樣本比對參數"=w248, "ROI Descriptor"=w268, "Mode"=w273, "error in (no error)"=w261, "Coordinate System In"=w267, "Template Image"=w278, "Image"=w254) -> ("error out"=w266:errorcluster, "Coordinate System Out"=w258:T14, "Matches (real-world)"=w272:T23)  [unwired: 1 in, 1 out]
                n96 = call "檢測_找邊_VI.vi"("Edge Options"=w255, "Scan Direction"=w257, "error in (no error)"=w266, "Coordinate System"=w258, "ROI"=w256, "Image"=w254) -> ("error out"=w265:errorcluster, "Array"=w251:cluster{"X":sgl, "Y":sgl}[])  [unwired: 3 in, 1 out]
                n97 = disable-structure shown="Enabled" {
                  disable-tunnel: w265 -> [w322 w325]
                  disable-tunnel: w259 -> [w321 w329]
                  disable-tunnel: w258 -> [w320 w327]
                  disable-tunnel: w254 -> [w316 w328]
                  disable-tunnel: [w315 w324] -> w253
                  disable-tunnel: [w314 _] -> w250
                  disable-tunnel: [_ w323] -> w243
                  frame Disabled {
                    n98 = Unbundle(w321) -> (w319:T6, w318:T22, w317)
                    n99 = call "檢測_找圓_VI.vi"("Edge Options"=w317, "Scan Direction"=w319, "error in (no error)"=w322, "Coordinate System"=w320, "ROI"=w318, "Image"=w316) -> ("error out"=w315:errorcluster, "Array"=w314:cluster{"X":sgl, "Y":sgl}[])  [unwired: 3 in, 1 out]
                  }
                  frame Enabled {
                    n100 = Unbundle(w329) -> ("ROI"=w326:T22)  [unwired: 1 out]
                    n101 = call "檢測_距離clamp_VI.vi"("error in (no error)"=w325, "Coordinate System"=w327, "ROI Descriptor"=w326, "Image"=w328) -> ("error out"=w324:errorcluster, "Distance"=w323:sgl)  [unwired: 4 in, 2 out]
                  }
                }
                n102 = Unbundle By Name(w248) -> ("分數"=w247:sgl)
                n103 = disable-structure shown="Enabled" {
                  disable-tunnel: w254 -> [w304 w307]
                  disable-tunnel: w253 -> [w303 _]
                  disable-tunnel: [w302 _] -> w252
                  disable-tunnel: w251 -> [w301 w309]
                  disable-tunnel: w250 -> [w300 _]
                  disable-tunnel: [_ w306] -> w245
                  disable-tunnel: [_ w305] -> w242
                  frame Disabled {
                    n104 = call "檢測_距離_VI.vi"("error in (no error)"=w303, "找圓"=w300, "找邊"=w301, "Image"=w304) -> ("error out"=w302:errorcluster, "min value"=→"彈簧距離":sgl)  [unwired: 4 in, 2 out]
                  }
                  frame Enabled {
                    n105 = Index Array(array=w309) -> (element=w308:cluster{"X":sgl, "Y":sgl})  [unwired: 1 in]
                    n106 = call "檢測_影像中心到邊距離.vi"("End Point"=w308, "Image"=w307) -> ("Distances"=w313:sgl[])  [unwired: 7 in, 2 out]
                    n107 = Index Array(array=w313) -> (element=w312:sgl)  [unwired: 1 in]
                    n108 = Divide(x=33.0, y=2592.0) -> (x/y=w305:dbl)
                    n109 = Multiply(x=w312, y=w305) -> (x*y=w306:dbl)
                  }
                }
                "距離(中心到邊)" <- w245
                n110 = Index Array(array=w272) -> (element=w271:T24)  [unwired: 1 in]
                n111 = Unbundle By Name(w271) -> ("Angle"=→"彈簧角度":sgl, "Score"=w249:sgl)
                n112 = Multiply(x=w243, y=w242) -> (x*y=→"間距":dbl)
              }
            }
            n113 = Greater Or Equal?(x=w199, y=w198) -> (x >= y?=w200:bool)
            n114 = Select(t=u32 6618880, s=w200, f=u32 16711680) -> (s? t:f=w206:u32)
            n115 = Select(t="OK", s=w200, f="NG") -> (s? t:f=→"String":string)
            n116 = property on="String" class="Str"("Text.TextColor"=w206, "Text.Size"=T13 {"Width"=160, "Height"=160}, "Text.FontSize"=u32 100 ("Text.Font:Size")) -> ()  [unwired: 2 in, 2 out]
          }
          frame Disabled {
            n117 = call "Image FGV.vi"("Image action"=Image_action."讀取圖片", "圖片名稱"="Image") -> ("Image Out"=w339:T1)  [unwired: 8 in, 1 out]
            n118 = property on="Image" class="ImageControl"() -> ("ROI"=w338:T22)  [unwired: 2 in, 2 out]
            n119 = call "IMAQ Find Circular Edge 3"("ROI Descriptor"=w338, "Image"=w339) -> ("Fitted Circle"=w336:T25, "Options"=w337:T26)  [unwired: 4 in, 4 out]
            n120 = Unbundle By Name(w336) -> ("Center (Pixels)"=w335:cluster{"X":sgl, "Y":sgl})
          }
        }
      }
      frame "             4.2.1浪代-Pattern" {
        n121 = local read "樣本比對參數L"() -> (w344:T3)
        n122 = property on="Image" class="ImageControl"() -> ("ROI"=w346:T22)  [unwired: 2 in, 2 out]
        n123 = call "Image FGV.vi"("Image action"=Image_action."讀取圖片", "圖片名稱"="Pattern") -> ("Image Out"=w347:T1)  [unwired: 8 in, 1 out]
        n124 = call "Image FGV.vi"("Image action"=Image_action."讀取圖片", "圖片名稱"="Image") -> ("Image Out"=w348:T1)  [unwired: 8 in, 1 out]
        n125 = Unbundle By Name(w344) -> ("方法"=w343:u16)
        n126 = To Long Integer(number=w343) -> (32bit integer=w342:i32)
        n127 = call "浪代_Pattern_Sub.vi"("Angle Range"="pattern_Angle Range", "Algorithm"=w342, "ROI"=w346, "Image Dst"=w347, "Image Src"=w348) -> ()  [unwired: 5 in, 2 out]
        n128 = Enqueue Element(queue=w357, element=Setting_Control_Main_Action."       3.2影像-更新影像", error in (no error)=w355) -> (queue out=w356:refnum<queue>, error out=w354:errorcluster)  [unwired: 1 in, 1 out]
      }
      frame "             4.2.2浪代-Match" {
        w384 = u16 0 items=["Find Reference", "Update CoordSys"] ("Mode")
        # "#Match FGV名稱\n塑膠Match-0\n彈簧Match-1\n以上皆使用相機數當名稱"
        n129 = property on="Image" class="ImageControl"() -> ("ROI"=w374:T22)  [unwired: 2 in, 2 out]
        n130 = call "Image FGV.vi"("Image action"=Image_action."讀取圖片", "圖片名稱"="Pattern") -> ("Image Out"=w383:T1)  [unwired: 8 in, 1 out]
        n131 = call "Image FGV.vi"("Image action"=Image_action."讀取圖片", "圖片名稱"="Image") -> ("Image Out"=w385:T1)  [unwired: 8 in, 1 out]
        n132 = call "浪代_Match_Sub.vi"("樣本比對參數"="樣本比對參數L", "ROI Descriptor"=w374, "Mode"=w384, "Coordinate System In"=T14 {"Reference System"={"Origin"={"X"=0.0, "Y"=0.0}, "Angle (deg)"=0.0, "Axis Reference"=0}, "Measurement System"={"Origin"={"X"=0.0, "Y"=0.0}, "Angle (deg)"=0.0, "Axis Reference"=0}}, "Template Image"=w383, "Image"=w385) -> ("error out"=w358:errorcluster, "Coordinate System Out"=w376:T14)  [unwired: 2 in, 2 out]
        n133 = local read "檢測項目塑膠蓋"() -> (w371:enum16{"Pattern", "Match", "找邊", "間距"})
        n134 = property on="檢測項目塑膠蓋" class="Enum (strict)"() -> ("Strings []"=w373:string[])  [unwired: 2 in, 2 out]
        n135 = To Long Integer(number=w371) -> (32bit integer=w372:i32)
        n136 = call "FGV_Indicator.vi"("Action"=Control_Indicator_Action(FGV)."Get Data") -> ("Indicator Data Out"=w366:T19)  [unwired: 10 in]
        n137 = Unbundle By Name(w366) -> ("相機、光源"=w365:cluster{"相機選擇":u8, "光源選擇":u16, "光源亮度":u8})
        n138 = Index Array(array=w373, index=w372) -> (element=w363:string)
        n139 = Bundle("樣本比對參數L"="樣本比對參數L", "ROI"=w374, "Coordinate System Out"=w376) -> (w369:T15)  [unwired: 1 in]
        n140 = To Variant(anything=w369) -> (Variant=w368:variant)
        n141 = Enqueue Element(queue=w381, element=Setting_Control_Main_Action."       3.2影像-更新影像", error in (no error)=w379) -> (queue out=w380:refnum<queue>, error out=w378:errorcluster)  [unwired: 1 in, 1 out]
        n142 = Unbundle By Name(w365) -> ("相機選擇"=w364:u8)
        n143 = Number To Decimal String(number=w364) -> (decimal integer string=w361:string)  [unwired: 1 in]
        n144 = Concatenate Strings(w363, "-" ("string"), w361) -> (w359:string)
        n145 = Bundle(w359, "Variant"=w368) -> (w360:cluster{string, "Variant":variant})  [unwired: 1 in]
        n146 = call "Main_FGV_Data.vi"("Action_Data"=Action_Data."Set Data", "Data In"=w360, "Data name"=w359) -> ()  [unwired: 7 in, 2 out]
        n147 = case shown="Error" w358 {
          frame No Error {
          }
          frame Error {
            n148 = One Button Dialog(message="match錯誤", button name ("OK")="確認") -> ()  [unwired: 1 out]
          }
        }
      }
      frame "             4.2.3檢測-找邊" {
        n149 = property on="Image" class="ImageControl"() -> ("ROI"=w403:T22)  [unwired: 2 in, 2 out]
        n150 = call "Image FGV.vi"("Image action"=Image_action."讀取圖片", "圖片名稱"="Image") -> ("error out"=w410:errorcluster, "Image Out"=w411:T1)  [unwired: 8 in]
        n151 = call "檢測_找邊_VI.vi"("Edge Options"="Edge Options", "Scan Direction"="Scan Direction", "error in (no error)"=w410, "Coordinate System"=T14 {"Reference System"={"Origin"={"X"=0.0, "Y"=0.0}, "Angle (deg)"=0.0, "Axis Reference"=0}, "Measurement System"={"Origin"={"X"=0.0, "Y"=0.0}, "Angle (deg)"=0.0, "Axis Reference"=0}}, "ROI"=w403, "Image"=w411) -> ("error out"=w392:errorcluster)  [unwired: 3 in, 2 out]
        n152 = local read "檢測項目塑膠蓋"() -> (w397:enum16{"Pattern", "Match", "找邊", "間距"})
        n153 = property on="檢測項目塑膠蓋" class="Enum (strict)"() -> ("Strings []"=w399:string[])  [unwired: 2 in, 2 out]
        n154 = Bundle("Scan Direction"="Scan Direction", "ROI"=w403, "Edge Options"="Edge Options") -> (w400:T18)  [unwired: 1 in]
        n155 = To Long Integer(number=w397) -> (32bit integer=w398:i32)
        n156 = To Variant(anything=w400) -> (Variant=w395:variant)
        n157 = Index Array(array=w399, index=w398) -> (element=w393:string)
        n158 = Bundle(w393, "Variant"=w395) -> (w394:cluster{string, "Variant":variant})  [unwired: 1 in]
        n159 = call "Main_FGV_Data.vi"("Action_Data"=Action_Data."Set Data", "Data In"=w394, "Data name"=w393) -> ()  [unwired: 7 in, 2 out]
        n160 = Enqueue Element(queue=w409, element=Setting_Control_Main_Action."       3.2影像-更新影像", error in (no error)=w408) -> (queue out=w407:refnum<queue>, error out=w406:errorcluster)  [unwired: 1 in, 1 out]
        n161 = case shown="Error" w392 {
          frame No Error {
          }
          frame Error {
            n162 = One Button Dialog(message="找邊錯誤", button name ("OK")="確認") -> ()  [unwired: 1 out]
          }
        }
      }
      frame "             4.2.4檢測-間距" {
        n163 = property on="Image" class="ImageControl"() -> ("ROI"=w416:T22)  [unwired: 2 in, 2 out]
        n164 = call "Image FGV.vi"("Image action"=Image_action."讀取圖片", "圖片名稱"="Image") -> ("Image Out"=w420:T1)  [unwired: 8 in, 1 out]
        n165 = disable-structure shown="Enabled" {
          disable-tunnel: w420 -> [w439 w444]
          disable-tunnel: w416 -> [w438 w443]
          disable-tunnel: T14 {"Reference System"={"Origin"={"X"=0.0, "Y"=0.0}, "Angle (deg)"=0.0, "Axis Reference"=0}, "Measurement System"={"Origin"={"X"=0.0, "Y"=0.0}, "Angle (deg)"=0.0, "Axis Reference"=0}} ("Coordinate System") -> [w437 w442]
          disable-tunnel: [w436 w441] -> w418
          disable-tunnel: [_ "setting"] -> w417
          frame Disabled {
            n166 = call "檢測_找圓_VI.vi"("Coordinate System"=w437, "ROI"=w438, "Image"=w439) -> ("error out"=w436:errorcluster)  [unwired: 6 in, 2 out]
          }
          frame Enabled {
            n167 = call "檢測_距離clamp_VI.vi"("setting"="setting", "Coordinate System"=w442, "ROI Descriptor"=w443, "Image"=w444) -> ("error out"=w441:errorcluster)  [unwired: 4 in, 3 out]
          }
        }
        n168 = local read "檢測項目塑膠蓋"() -> (w425:enum16{"Pattern", "Match", "找邊", "間距"})
        n169 = property on="檢測項目塑膠蓋" class="Enum (strict)"() -> ("Strings []"=w427:string[])  [unwired: 2 in, 2 out]
        n170 = Bundle("setting"=w417, "ROI"=w416) -> (w428:T17)  [unwired: 1 in]
        n171 = To Long Integer(number=w425) -> (32bit integer=w426:i32)
        n172 = To Variant(anything=w428) -> (Variant=w423:variant)
        n173 = Index Array(array=w427, index=w426) -> (element=w421:string)
        n174 = Bundle(w421, "Variant"=w423) -> (w422:cluster{string, "Variant":variant})  [unwired: 1 in]
        n175 = call "Main_FGV_Data.vi"("Action_Data"=Action_Data."Set Data", "Data In"=w422, "Data name"=w421) -> ()  [unwired: 7 in, 2 out]
        n176 = case shown="Error" w418 {
          frame No Error {
          }
          frame Error {
            n177 = One Button Dialog(message="間距錯誤", button name ("OK")="確認") -> ()  [unwired: 1 out]
          }
        }
        n178 = Enqueue Element(queue=w435, element=Setting_Control_Main_Action."       3.2影像-更新影像", error in (no error)=w434) -> (queue out=w433:refnum<queue>, error out=w432:errorcluster)  [unwired: 1 in, 1 out]
      }
      frame "5.0功能-檔案" {
      }
      frame "       5.1檔案-初始化" {
        n179 = call "Main_FGV_Data.vi"("Action_Data"=Action_Data."Initialize") -> ()  [unwired: 9 in, 2 out]
      }
      frame "       5.2檔案-儲存檔案" {
        # "#儲存檔案\n看此資料夾裡是否有東西\n有的話就砍掉，沒有就直接儲存"
        n180 = call "FGV_Indicator.vi"("Action"=Control_Indicator_Action(FGV)."Get Data") -> ("Indicator Data Out"=w462:T19)  [unwired: 10 in]
        n181 = Unbundle By Name(w462) -> ("Cam#Light#Strength"=w453:string)
        n182 = Unbundle By Name(w462) -> ("相機、光源"=w461:cluster{"相機選擇":u8, "光源選擇":u16, "光源亮度":u8})
        n183 = Unbundle By Name(w461) -> ("相機選擇"=w460:u8)
        n184 = case shown="0, Default" w460 {
          tunnel: ["CCD1-塑膠" "CCD2-彈簧"] -> w458
          frame 0, Default {
          }
          frame 1 {
          }
        }
        n185 = Build Path(base path=path "D:/渦輪組裝機參數/Data 資料/Setting Data" ("file (use dialog)"), name or relative path=w458) -> (appended path=w455:path)
        n186 = File/Directory Info(path=w455) -> (size=w457:i64)  [unwired: 1 in, 6 out]
        n187 = Equal To 0?(x=w457) -> (x = 0?=w456:bool)
        n188 = case shown="False" w456 {
          tunnel: w455 -> [w475 w480]
          tunnel: [w475 w480] -> w454
          frame False {
            n189 = List Folder(path=w475) -> (filenames=w476:string[])  [unwired: 3 in, 3 out]
            n190 = for {
              tunnel: w476 -> [w478] mode=indexing
              tunnel: w475 -> [w479]
              n191 = Build Path(base path=w479, name or relative path=w478) -> (appended path=w477:path)
              n192 = Delete(path (use dialog)=w477) -> ()  [unwired: 4 in, 3 out]
            }
          }
          frame True {
          }
        }
        n193 = call "Main_FGV_Data.vi"("Action_Data"=Action_Data."Idle") -> ("Data Array out"=w471:cluster{"Data name":string, "Data":variant}[])  [unwired: 9 in, 1 out]
        n194 = call "Image FGV.vi"("Image action"=Image_action."讀取圖片", "圖片名稱"="Pattern") -> ("Image Out"=w468:T1)  [unwired: 8 in, 1 out]
        n195 = Concatenate Strings(w453, ".png" ("string")) -> (w463:string)
        n196 = Build Path(base path=w454, name or relative path=w453) -> (appended path=w470:path)
        n197 = Build Path(base path=w454, name or relative path=w463) -> (appended path=w466:path)
        n198 = Write to Binary File(file (use dialog)=w470, data=w471) -> (error out=w467:errorcluster)  [unwired: 4 in, 2 out]
        n199 = call "IMAQ Write Image And Vision Info File 2"("error in (no error)"=w467, "File Path"=w466, "Image"=w468) -> ()  [unwired: 7 in, 2 out]
      }
      frame "       5.3檔案-開啟檔案" {
        # "#開啟檔案\n錯誤表示沒有開檔，並\n強制設為CCD1取像\n沒有錯誤表示有開檔"
        n200 = call "File Dialog"("start path"=path "D:/渦輪組裝機參數/Data 資料/Setting Data") -> ("selected path"=w488:path, "error out"=w504:errorcluster)  [unwired: 11 in, 2 out]
        n201 = Strip Path(path=w488) -> (stripped path=w485:path, name=w487:string)
        n202 = Concatenate Strings(w487, ".png" ("string")) -> (w484:string)
        n203 = Build Path(base path=w485, name or relative path=w484) -> (appended path=w483:path)
        n204 = call "Main_FGV_Data.vi"("Action_Data"=Action_Data."Idle") -> ("Data Array out"=w502:cluster{"Data name":string, "Data":variant}[])  [unwired: 9 in, 1 out]
        n205 = Read from Binary File(5:w502, 8:w504, 11:w488) -> (0:w496:errorcluster, 2:w501:cluster{"Data name":string, "Data":variant}[])  [unwired: 3 in, 2 out]
        n206 = call "Image FGV.vi"("Image action"=Image_action."讀取圖片", "error in (no error)"=w496, "圖片名稱"="Pattern") -> ("error out"=w495:errorcluster, "Image Out"=w497:T1)  [unwired: 7 in]
        n207 = call "IMAQ Read Image And Vision Info"("File Path"=w483, "error in (no error)"=w495, "Image"=w497) -> ("error out"=w489:errorcluster)  [unwired: 6 in, 2 out]
        n208 = case shown="Error" w496 {
          tunnel: w488 -> [w505 _]
          frame No Error {
            n209 = Strip Path(path=w505) -> (name=w507:string)  [unwired: 1 out]
            n210 = call "SubVI_Cam&Li_String.vi"("Data String In"=w507) -> ("相機、光源"=w509:T2)  [unwired: 10 in]
            n211 = Bundle By Name(cluster=T19 {"相機、光源"={"相機選擇"=0, "光源選擇"=0, "光源亮度"=0}, "Session Out"="cam0", "Cam#Light#Strength"="CCD11126"} ("Indicator Data In"), "相機、光源"=w509) -> (w510:T19)
            n212 = call "FGV_Indicator.vi"("Action"=Control_Indicator_Action(FGV)."Set Data", "Indicator Data In"=w510) -> ()  [unwired: 9 in, 1 out]
          }
          frame Error {
            n213 = Bundle By Name(cluster=T19 {"相機、光源"={"相機選擇"=0, "光源選擇"=0, "光源亮度"=0}, "Session Out"="cam0", "Cam#Light#Strength"=""} ("Indicator Data In"), "相機、光源"=cluster{"相機選擇":u8, "光源選擇":u16, "光源亮度":u8} {"相機選擇"=0, "光源選擇"=0, "光源亮度"=0}) -> (w512:T19)
            n214 = call "FGV_Indicator.vi"("Action"=Control_Indicator_Action(FGV)."Set Data", "Indicator Data In"=w512) -> ()  [unwired: 9 in, 1 out]
          }
        }
        n215 = for {
          tunnel: w501 -> [w515] mode=indexing
          tunnel: w496 -> [_]
          n216 = Unbundle(w515) -> ("Data name"=w516:string)  [unwired: 1 out]
          n217 = call "Main_FGV_Data.vi"("Action_Data"=Action_Data."Set Data", "Data In"=w515, "Data name"=w516) -> ()  [unwired: 7 in, 2 out]
        }
        n218 = Enqueue Element(queue=w493, element=Setting_Control_Main_Action."       3.2影像-更新影像", error in (no error)=w492) -> (queue out=w494:refnum<queue>, error out=w491:errorcluster)  [unwired: 1 in, 1 out]
      }
      frame "       5.4檔案-匯入檔案" {
        # "#匯入檔案\n有錯誤表示沒有匯入檔案所以給常數\n沒錯誤表示有匯入檔案直接給儲存參數"
        n219 = property on="檢測項目塑膠蓋" class="Enum (strict)"() -> ("Strings []"=w539:string[])  [unwired: 2 in, 2 out]
        n220 = To Long Integer(number=enum16{"Pattern", "Match", "找邊", "間距"}."間距" ("檢測項目塑膠蓋")) -> (32bit integer=w541:i32)
        n221 = To Long Integer(number=enum16{"Pattern", "Match", "找邊", "間距"}."找邊" ("檢測項目塑膠蓋")) -> (32bit integer=w550:i32)
        n222 = Index Array(array=w539, index=w541) -> (element=w534:string)
        n223 = call "FGV_Indicator.vi"("Action"=Control_Indicator_Action(FGV)."Get Data") -> ("Indicator Data Out"=w561:T19)  [unwired: 10 in]
        n224 = Index Array(array=w539, index=w550) -> (element=w535:string)
        n225 = To Long Integer(number=enum16{"Pattern", "Match", "找邊", "間距"}."Match" ("檢測項目塑膠蓋")) -> (32bit integer=w558:i32)
        n226 = Unbundle By Name(w561) -> ("相機、光源"=w553:cluster{"相機選擇":u8, "光源選擇":u16, "光源亮度":u8})
        n227 = Index Array(array=w539, index=w558) -> (element=w537:string)
        n228 = local write "相機、光源"(w553) -> ()
        n229 = Unbundle By Name(w553) -> ("相機選擇"=w538:u8)
        n230 = Number To Decimal String(number=w538) -> (decimal integer string=w552:string)  [unwired: 1 in]
        n231 = Concatenate Strings(w537, "-" ("string"), w552) -> (w536:string)
        n232 = Build Array(w536, w535, w534) -> (w533:string[])
        n233 = for {
          tunnel: w533 -> [w568] mode=indexing
          tunnel: [w567] -> w532 mode=indexing
          n234 = call "Main_FGV_Data.vi"("Action_Data"=Action_Data."Get Data", "Data name"=w568) -> ("Data  Out"=w567:cluster{"Data name":string, "Data":variant})  [unwired: 8 in, 1 out]
        }
        n235 = case shown="1" w538 {
          frame 0, Default {
            n236 = property on="檢測項目塑膠蓋" class="Enum (strict)"("Disabled Items []"=i32[] [2, 3]) -> ()  [unwired: 2 in, 2 out]
          }
          frame 1 {
            n237 = property on="檢測項目塑膠蓋" class="Enum (strict)"("Disabled Items []"=i32[] []) -> ()  [unwired: 2 in, 2 out]
          }
        }
        n238 = Index Array(array=w532, index #1=0 ("index"), index #2=1 ("index"), index #3=2 ("index")) -> (element #1=w528:cluster{"Data name":string, "Data":variant}, element #2=w527:cluster{"Data name":string, "Data":variant}, element #3=w526:cluster{"Data name":string, "Data":variant})
        n239 = Unbundle By Name(w526) -> ("Data"=w540:variant)
        n240 = Unbundle By Name(w528) -> ("Data"=w560:variant)
        n241 = Unbundle By Name(w527) -> ("Data"=w549:variant)
        n242 = Variant To Data(type=T17 {"setting"={"Contrast"=0, "Filter width"=0, "Steepness"=0, "Subsampling Ratio"=0}, "ROI"={"Global Rectangle"=[], "Contours"=[]}} ("output cluster"), Variant=w540) -> (data=w520:T17, error out=w525:errorcluster)  [unwired: 1 in]
        n243 = Variant To Data(type=T18 {"Scan Direction"=0, "ROI"={"Global Rectangle"=[], "Contours"=[]}, "Edge Options"={"Edge Polarity"=0, "Kernel Size"=0, "Width"=0, "Minimum Edge Strength"=0.0, "Interpolation Type"=enum."Zero Order", "Data Processing Method"=enum."Average"}} ("output cluster"), Variant=w549) -> (data=w547:T18, error out=w546:errorcluster)  [unwired: 1 in]
        n244 = Variant To Data(type=T15 {"樣本比對參數L"={"方法"=0, "分數"=0.0, "起始角度"=0.0, "結束角度"=0.0}, "ROI"={"Global Rectangle"=[], "Contours"=[]}, "Coordinate System Out"={"Reference System"={"Origin"={"X"=0.0, "Y"=0.0}, "Angle (deg)"=0.0, "Axis Reference"=0}, "Measurement System"={"Origin"={"X"=0.0, "Y"=0.0}, "Angle (deg)"=0.0, "Axis Reference"=0}}} ("output cluster"), Variant=w560) -> (data=w557:T15, error out=w556:errorcluster)  [unwired: 1 in]
        n245 = Unbundle By Name(w520) -> ("setting"=w519:T6)
        n246 = Unbundle By Name(w547) -> ("Scan Direction"=w545:u16, "Edge Options"=w543:T4)
        n247 = Unbundle By Name(w557) -> ("樣本比對參數L"=w555:T3)
        n248 = case shown="No Error" w546 {
          tunnel: [w571 u16 0 ("Scan Direction")] -> w544
          tunnel: w545 -> [w571 _]
          tunnel: w543 -> [w570 _]
          tunnel: [w570 T4 {"Edge Polarity"=0, "Kernel Size"=3, "Width"=3, "Minimum Edge Strength"=10.0, "Interpolation Type"=enum."Bilinear Fixed", "Data Processing Method"=enum."Average"} ("Edge Options")] -> w542
          frame No Error {
          }
          frame Error {
          }
        }
        n249 = case shown="Error" w525 {
          tunnel: w519 -> [w565 _]
          tunnel: [w565 T6 {"Contrast"=40, "Filter width"=4, "Steepness"=2, "Subsampling Ratio"=5} ("setting")] -> w518
          frame No Error {
          }
          frame Error {
          }
        }
        n250 = case shown="No Error" w556 {
          tunnel: w555 -> [w576 _]
          tunnel: [w576 T3 {"方法"=1, "分數"=800.0, "起始角度"=-5.0, "結束角度"=5.0} ("樣本比對參數L")] -> w554
          frame No Error {
          }
          frame Error {
          }
        }
        n251 = local write "setting"(w518) -> ()
        n252 = local write "Scan Direction"(w544) -> ()
        n253 = local write "Edge Options"(w542) -> ()
        n254 = local write "樣本比對參數L"(w554) -> ()
      }
      frame "6.0 錯誤" {
      }
      frame "7.0等待" {
      }
      frame "       7.1等待(計算時間)" {
      }
      frame "8.0離開" {
      }
      frame "9.0功能-機台驗證" {
      }
      frame "      9.1機台驗證-初始化" {
      }
      frame "      9.2機台驗證-檢測" {
      }
      frame "10.0對話視窗" {
      }
      frame "11.光源控制" {
      }
      frame "       11.1光源控制-初始化" {
        n255 = disable-structure shown="Disabled" {
          frame Disabled {
            n256 = call "RS232 Device.vi"() -> ("error out"=w599:errorcluster, "COM"=w600:refnum<visa-resource-name>)  [unwired: 10 in]
            n257 = call "光源通訊_FGV.vi"("通訊_action"=光源通訊_action_control."initial", "error in (no error)"=w599, "VISA resource name"=w600) -> ()  [unwired: 7 in, 2 out]
          }
          frame Enabled {
          }
        }
      }
      frame "       11.2光源控制-光源開啟" {
        n258 = call "FGV_Indicator.vi"("Action"=Control_Indicator_Action(FGV)."Get Data") -> ("Indicator Data Out"=w608:T19)  [unwired: 10 in]
        n259 = Unbundle By Name(w608) -> ("相機、光源"=w607:cluster{"相機選擇":u8, "光源選擇":u16, "光源亮度":u8})
        n260 = Unbundle By Name(w607) -> ("光源選擇"=w605:u16, "光源亮度"=w606:u8)
        n261 = To Unsigned Byte Integer(number=w605) -> (unsigned 8bit integer=w604:u8)
        n262 = Increment(x=w604) -> (x+1=w603:u8)
        n263 = call "光源通訊_FGV.vi"("通訊_action"=光源通訊_action_control."開啟光源", "亮度"=w606, "通道"=w603) -> ("error out"=w602:errorcluster)  [unwired: 7 in, 1 out]
        n264 = case shown="Error" w602 {
          frame No Error {
          }
          frame Error {
            n265 = One Button Dialog(message="光源開啟錯誤", button name ("OK")="確認") -> ()  [unwired: 1 out]
          }
        }
      }
      frame "       11.3光源控制-光源關閉" {
        n266 = call "FGV_Indicator.vi"("Action"=Control_Indicator_Action(FGV)."Get Data") -> ("Indicator Data Out"=w620:T19)  [unwired: 10 in]
        n267 = Unbundle By Name(w620) -> ("相機、光源"=w619:cluster{"相機選擇":u8, "光源選擇":u16, "光源亮度":u8})
        n268 = Unbundle By Name(w619) -> ("光源選擇"=w618:u16)  [unwired: 1 out]
        n269 = To Unsigned Byte Integer(number=w618) -> (unsigned 8bit integer=w617:u8)
        n270 = Increment(x=w617) -> (x+1=w616:u8)
        n271 = call "光源通訊_FGV.vi"("通訊_action"=光源通訊_action_control."關閉光源", "通道"=w616) -> ("error out"=w615:errorcluster)  [unwired: 8 in, 1 out]
        n272 = case shown="Error" w615 {
          frame No Error {
          }
          frame Error {
            n273 = One Button Dialog(message="光源關閉錯誤", button name ("OK")="確認") -> ()  [unwired: 1 out]
          }
        }
      }
      frame "       11.4光源控制-通訊關閉" {
        n274 = disable-structure shown="Disabled" {
          frame Disabled {
            n275 = call "光源通訊_FGV.vi"("通訊_action"=光源通訊_action_control."close") -> ()  [unwired: 9 in, 2 out]
          }
          frame Enabled {
          }
        }
      }
    }
  }
  n276 = while {
    tunnel: w6 -> [w635]
    tunnel: w5 -> [w634]
    stop <- w633 stop-if-true
    n277 = event shown="[5] \"檢測項目塑膠蓋\": Value Change" {
      selector: _ -> [_ _ _ _ _ _ _ _ _]
      dyn-events: _ -> [_ _ _ _ _ _ _ _ _]
      timeout: _ -> [_ _ _ _ _ _ _ _ _]
      tunnel: w635 -> [w637 w640 w654 w661 w666 w682 w685 w688 w691]
      tunnel: [w637 w640 w654 w661 w665 w682 w685 w688 w691] -> w632
      tunnel: w634 -> [w636 w639 w653 w660 w664 w681 w684 w687 w690]
      tunnel: [w636 w639 w653 w660 w663 w681 w684 w687 w690] -> w631
      tunnel: [_ _ _ _ _ _ _ _ TRUE] -> w633
      tunnel: [_ Setting_Control_Main_Action."二、動作-單次取像" ("Set action") Setting_Control_Main_Action."       7.1等待(計算時間)" ("Set action") Setting_Control_Main_Action."三、動作-連續取像" ("Set action") w662 Setting_Control_Main_Action."       7.1等待(計算時間)" ("Set action") Setting_Control_Main_Action."四、動作-單步測試" ("Set action") Setting_Control_Main_Action."五、動作-連續測試" ("Set action") Setting_Control_Main_Action."六、動作-離開" ("Set action")] -> w630
      event Timeout {
        n278 = event-data() -> ()  [unwired: 1 in, 3 out]
      }
      event "取像": Value Change {
        n279 = event-data() -> ()  [unwired: 1 in, 1 out]
      }
      event Value Change {
        n280 = event-data() -> ()  [unwired: 1 in, 1 out]
        n281 = Bundle By Name(cluster=T19 {"相機、光源"={"相機選擇"=0, "光源選擇"=0, "光源亮度"=0}, "Session Out"="cam0", "Cam#Light#Strength"=""} ("Indicator Data In"), "相機、光源"="相機、光源") -> (w649:T19)
        n282 = Unbundle By Name("相機、光源") -> ("相機選擇"=w647:u8, "光源選擇"=w645:u16, "光源亮度"=w644:u8)
        n283 = case shown="1" w647 {
          frame 0, Default {
            n284 = property on="檢測項目塑膠蓋" class="Enum (strict)"("Disabled Items []"=i32[] [2, 3]) -> ()  [unwired: 2 in, 2 out]
          }
          frame 1 {
            n285 = property on="檢測項目塑膠蓋" class="Enum (strict)"("Disabled Items []"=i32[] []) -> ()  [unwired: 2 in, 2 out]
          }
        }
        n286 = call "FGV_Indicator.vi"("Action"=Control_Indicator_Action(FGV)."Set Data", "Indicator Data In"=w649) -> ()  [unwired: 9 in, 1 out]
        n287 = To Unsigned Byte Integer(number=w645) -> (unsigned 8bit integer=w643:u8)
        n288 = Increment(x=w643) -> (x+1=w642:u8)
        n289 = call "光源通訊_FGV.vi"("通訊_action"=光源通訊_action_control."開啟光源", "亮度"=w644, "通道"=w642) -> ("error out"=w641:errorcluster)  [unwired: 7 in, 1 out]
        n290 = case shown="Error" w641 {
          frame No Error {
          }
          frame Error {
            n291 = One Button Dialog(message="光源開啟錯誤", button name ("OK")="確認") -> ()  [unwired: 1 out]
          }
        }
      }
      event "連續取像": Value Change {
        n292 = event-data() -> ()  [unwired: 1 in, 1 out]
      }
      event "確認檢測項目": Value Change {
        n293 = event-data() -> ()  [unwired: 1 in, 1 out]
        n294 = local read "檢測項目塑膠蓋"() -> (w667:enum16{"Pattern", "Match", "找邊", "間距"})
        n295 = case shown="\"間距\"" w667 {
          tunnel: w666 -> [w670 w673 w676 w679]
          tunnel: [w670 w673 w676 w679] -> w665
          tunnel: w664 -> [w669 w672 w675 w678]
          tunnel: [w669 w672 w675 w678] -> w663
          tunnel: [Setting_Control_Main_Action."             4.2.1浪代-Pattern" ("Set action") Setting_Control_Main_Action."             4.2.2浪代-Match" ("Set action") Setting_Control_Main_Action."             4.2.3檢測-找邊" ("Set action") Setting_Control_Main_Action."             4.2.4檢測-間距" ("Set action")] -> w662
          frame "Pattern", Default {
          }
          frame "Match" {
          }
          frame "找邊" {
          }
          frame "間距" {
          }
        }
      }
      event "檢測項目塑膠蓋": Value Change {
        n296 = event-data() -> ()  [unwired: 1 in, 2 out]
      }
      event "單步測試": Value Change {
        n297 = event-data() -> ()  [unwired: 1 in, 1 out]
      }
      event "連續測試": Value Change {
        n298 = event-data() -> ()  [unwired: 1 in, 1 out]
      }
      event "離開": Value Change {
        n299 = event-data() -> ()  [unwired: 1 in, 1 out]
      }
    }
    n300 = Enqueue Element(queue=w632, element=w630, error in (no error)=w631) -> ()  [unwired: 1 in, 3 out]
  }
  n301 = Release Queue(queue=w2, error in (no error)=w1) -> ()  [unwired: 1 in, 3 out]
